vi "search for hook (1).vi"(10 "RobotDriveDevRef in":T1, 11 "Hook Found":bool) -> (0 "error out":errorcluster, 1 "Pixels to turn":dbl, 2 "RobotDriveDevRef out":T1, 3 "Move forward? S 5":bool, 4 "Hook found":bool, 5 "Hook Found In False Case 2":bool, 6 "Degrees to turn":dbl, 7 "Hook Center":dbl)   [LabVIEW 2016]
uses:
  <vilib>/Rock Robotics/WPI/RobotDrive/WPI_RobotDriveDevRef.ctl
  <vilib>/Rock Robotics/WPI/MotorControl/WPI_MotorControlDeviceRef.ctl
  <vilib>/Rock Robotics/WPI/MotorControl/WPI_MotorControlType.ctl
  <vilib>/Rock Robotics/SystemInterfaces/DIO/FPGA_DIOPWMChannel.ctl
  <vilib>/Rock Robotics/WPI/PWM/WPI_PWMDeadband.ctl
  <vilib>/Rock Robotics/Network Tables/NT Write Number.vi
  Robot Global Data.vi
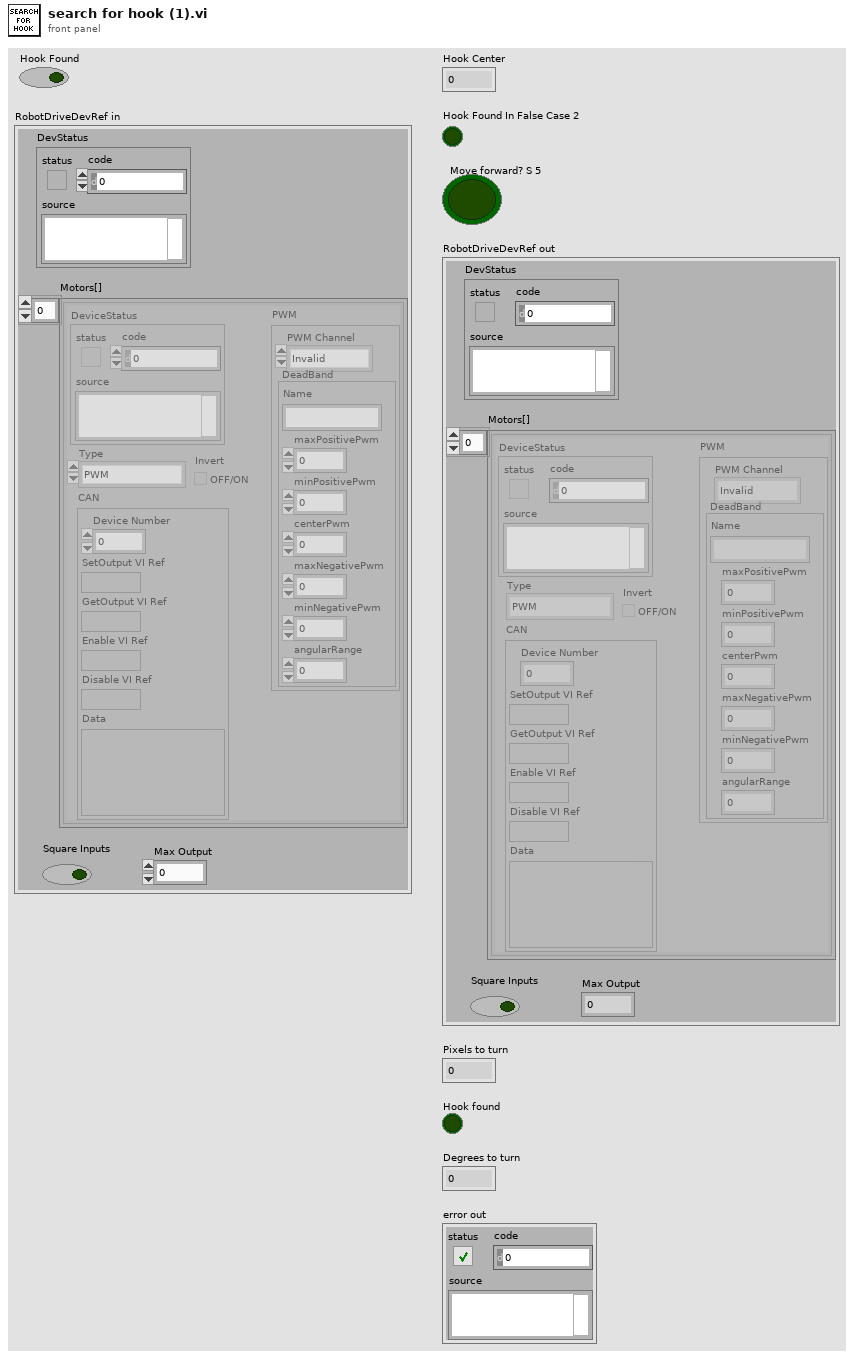
[diagram p1: front panel]
types:
  T1 = typedef "WPI_RobotDriveDevRef.ctl" = cluster{"DevStatus":errorcluster, "Motors[]":T2[], "Square Inputs":bool, "Max Output":dbl}
  T2 = typedef "WPI_MotorControlDeviceRef.ctl" = cluster{"DeviceStatus":errorcluster, "Type":T3, "PWM":cluster{"PWM Channel":T4, "DeadBand":T5}, "CAN":cluster{"Device Number":u8, "SetOutput VI Ref":variant, "GetOutput VI Ref":variant, "Enable VI Ref":variant, "Disable VI Ref":variant, "Data":variant}, "Invert":bool}
  T3 = typedef "WPI_MotorControlType.ctl" = enum16{"PWM", "CAN"}
  T4 = typedef "FPGA_DIOPWMChannel.ctl" = enum8{"PWM 0", "PWM 1", "PWM 2", "PWM 3", "PWM 4", "PWM 5", "PWM 6", "PWM 7", "PWM 8", "PWM 9", "PWM MXP 0", "PWM MXP 1", "PWM MXP 2", "PWM MXP 3", "PWM MXP 4", "PWM MXP 5", "PWM MXP 6", "PWM MXP 7", "PWM MXP 8", "PWM MXP 9", "Invalid"}
  T5 = typedef "WPI_PWMDeadband.ctl" = cluster{"Name":string, "maxPositivePwm":i32, "minPositivePwm":i32, "centerPwm":i32, "maxNegativePwm":i32, "minNegativePwm":i32, "angularRange":u16}
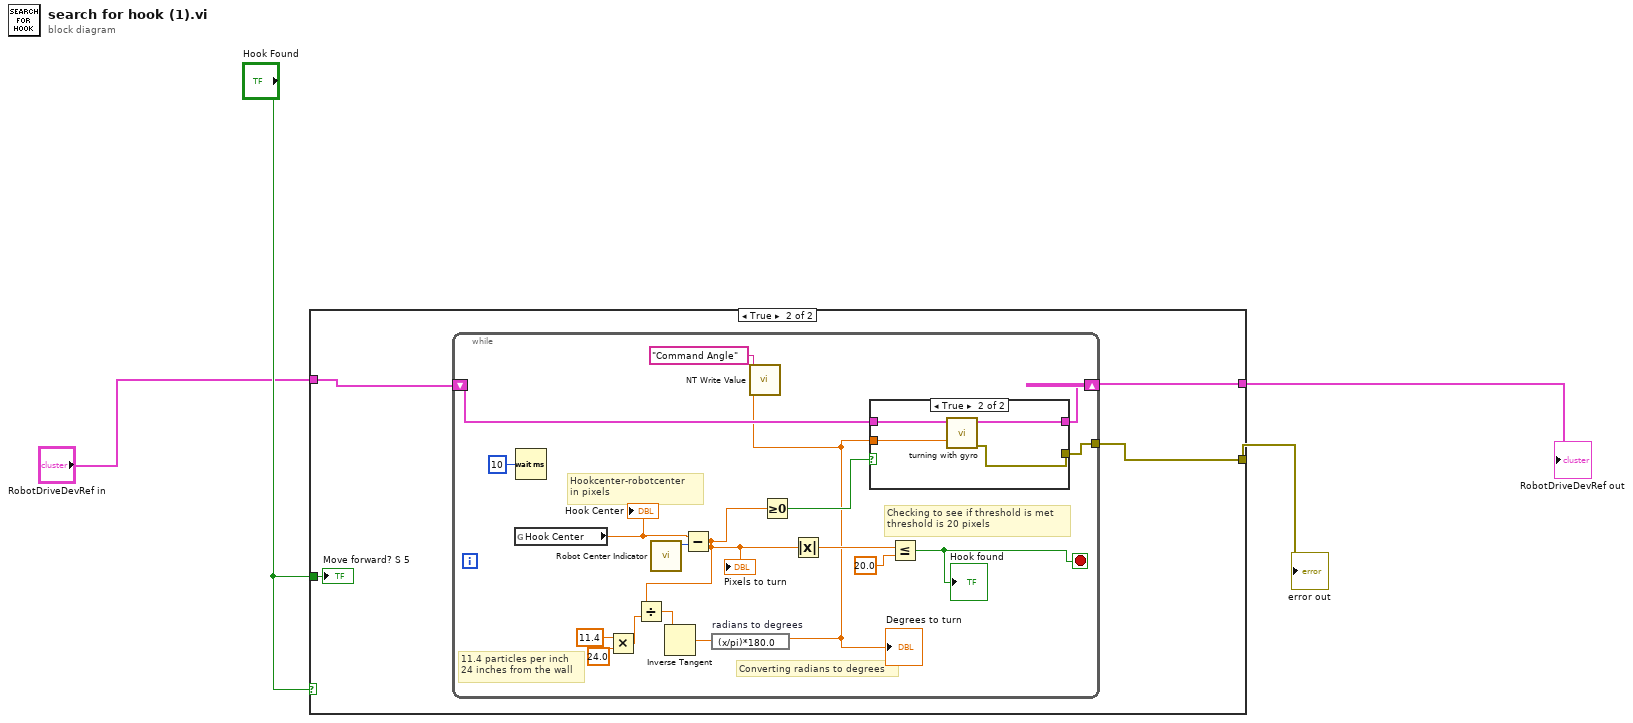
[diagram p0: block diagram]
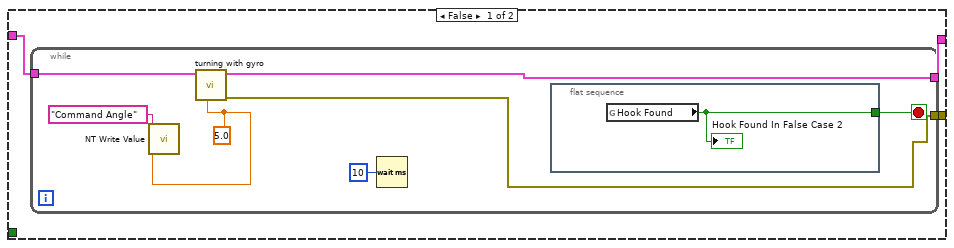
[diagram p2: hidden frame]
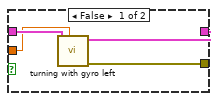
[diagram p3: hidden frame]
diagram:
  n1 = case shown="True" "Hook Found" {
    tunnel: [w7 w19] -> w3
    tunnel: "RobotDriveDevRef in" -> [w6 w18]
    tunnel: [w5 w17] -> w2
    tunnel: "Hook Found" -> [_ w16]
    frame False {
      n2 = while {
        tunnel: [w13] -> w7
        tunnel: w6 -> [w12]
        tunnel: [w11] -> w5
        stop <- w14 stop-if-true
        w9 = 5.0 ("desired angle")
        n3 = call-poly <vilib>:"NT Write Value.vi"("Numeric"=w9, "Name"="Command Angle") -> ()  [unwired: 9 in, 1 out]
        n4 = call "turning with gyro.vi"("desired angle"=w9, "RobotDriveDevRef"=w12) -> ("error out"=w11:errorcluster, "RobotDriveDevRef 2"=w13:T1)  [unwired: 8 in]
        n5 = Wait (ms)(milliseconds to wait=u32 10) -> ()  [unwired: 1 out]
        n6 = flat-sequence {
          tunnel: [w15] -> w14
          frame #0 {
            n7 = global read "Robot Global Data.vi" "Hook Found"() -> (w15:bool)
            "Hook Found In False Case 2" <- w15
          }
        }
      }
    }
    frame True {
      n8 = while {
        shift-right: [w33] -> w19
        shift-left: w18 -> [w34]
        tunnel: [w23] -> w17
        stop <- w24 stop-if-true
        # "Checking to see if threshold is met\nthreshold is 20 pixels"
        # "Hookcenter-robotcenter \nin pixels"
        # "11.4 particles per inch\n24 inches from the wall"
        # "Converting radians to degrees"
        n9 = global read "Robot Global Data.vi" "Hook Center"() -> (w36:dbl)
        "Hook Center" <- w36
        n10 = Wait (ms)(milliseconds to wait=u32 10) -> ()  [unwired: 1 out]
        n11 = Multiply(x=11.4, y=24.0) -> (x*y=w28:dbl)
        n12 = call "Robot Center Indicator.vi"() -> ("Robot Center"=w37:i32)  [unwired: 10 in, 1 out]
        n13 = Subtract(x=w36, y=w37) -> (x-y=w25:dbl)
        "Pixels to turn" <- w25
        n14 = Divide(x=w25, y=w28) -> (x/y=w29:dbl)
        n15 = Inverse Tangent(1:w29) -> (0:w30:dbl)
        n16 = expression code="(x/pi)*180.0" "radians to degrees"(w30) -> (w21:dbl)
        "Degrees to turn" <- w21
        n17 = call-poly <vilib>:"NT Write Value.vi"("Numeric"=w21, "Name"="Command Angle") -> ()  [unwired: 9 in, 1 out]
        n18 = Greater Or Equal To 0?(x=w25) -> (x >= 0?=w35:bool)
        n19 = Absolute Value(x=w25) -> (abs(x)=w32:dbl)
        n20 = case shown="True" w35 {
          tunnel: w34 -> [w41 w45]
          tunnel: [w40 w44] -> w33
          tunnel: w21 -> [w39 w43]
          tunnel: [w38 w42] -> w23
          frame False {
            n21 = call "turning with gyro left.vi"("desired angle"=w39, "RobotDriveDevRef"=w41) -> ("error out"=w38:errorcluster, "RobotDriveDevRef 2"=w40:T1)  [unwired: 8 in]
          }
          frame True {
            n22 = call "turning with gyro.vi"("desired angle"=w43, "RobotDriveDevRef"=w45) -> ("error out"=w42:errorcluster, "RobotDriveDevRef 2"=w44:T1)  [unwired: 8 in]
          }
        }
        n23 = Less Or Equal?(x=w32, y=20.0) -> (x <= y?=w24:bool)
        "Hook found" <- w24
      }
      "Move forward? S 5" <- w16
    }
  }
  "RobotDriveDevRef out" <- w3
  "error out" <- w2
